vi "Publish.vi"(6 "Publish Time":timestamp, 8 "error in (no error)":errorcluster, 9 "Data to Publish":variant, 10 "Datum Name":string, 11 "Mediator in":refnum<class "Mediator.lvclass">) -> (0 "error out":errorcluster, 3 "Mediator out":refnum<class "Mediator.lvclass">)   [LabVIEW 2015, in "Mediator.lvlib" / "Mediator.lvclass"]
doc: "<License>\nCopyright © 2017 Composed Systems, LLC | All rights reserved\nwww.composed.io\n\nAuthor: Ethan Stern <ethan.stern@composed.io>\n\nThis software is provided \"AS IS\" WITHOUT WARRANTIES, either express or implied, AND IS FOR EDUCATIONAL PURPOSES ONLY.\n</License>"
uses:
  Mediator.lvclass
  Mediator.lvclass/Mediator.ctl
  Topic Messages/Notify Subscribers Msg/Notify Subscribers Msg.lvclass/Notify Subscribers Msg.ctl
  <vilib>/ActorFramework/Message Enqueuer/Message Enqueuer.lvclass/Message Enqueuer.ctl
  <vilib>/ActorFramework/Message Enqueuer/Enqueue.vi
  <vilib>/ActorFramework/Message Priority Queue/Priority Enqueue.vi
  Topic Messages/Notify Subscribers Msg/Notify Subscribers Msg.lvclass
  TopicLookupTable/TopicLookupTable.lvclass
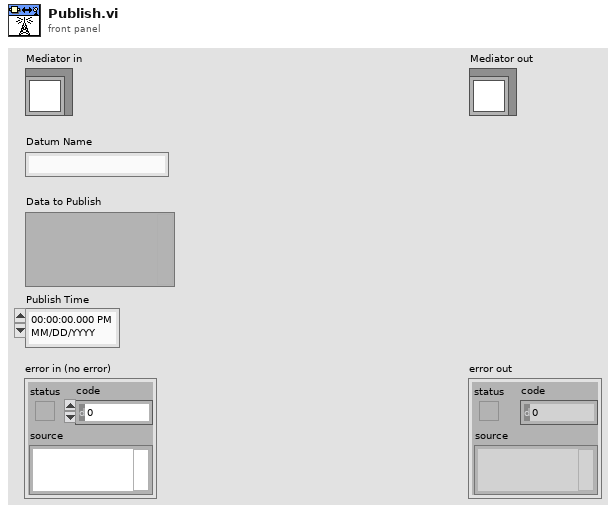
[diagram p1: front panel]
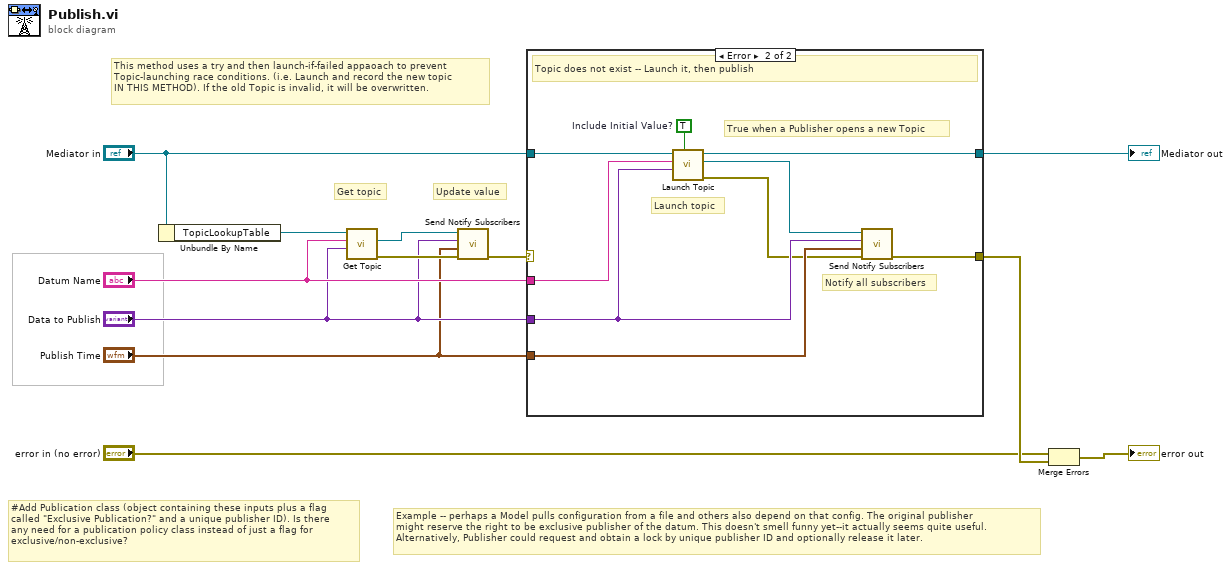
[diagram p0: block diagram]
diagram:
  # "Example -- perhaps a Model pulls configuration from a file and others also depend on that config. The original publisher\nmight reserve the right to be exclusive publisher of the datum. This doesn't smell funny yet--it actually seems quite useful.\nAlternatively, Publisher could request and obtain a lock by unique publisher ID and optionally release it later."
  # "#Add Publication class (object containing these inputs plus a flag \ncalled \"Exclusive Publication?\" and a unique publisher ID). Is there\nany need for a publication policy class instead of just a flag for\nexclusive/non-exclusive?"
  # "This method uses a try and then launch-if-failed appaoach to prevent\nTopic-launching race conditions. (i.e. Launch and record the new topic\nIN THIS METHOD). If the old Topic is invalid, it will be overwritten."
  # "Update value"
  # "Get topic"
  n1 = Unbundle By Name("Mediator in") -> ("TopicLookupTable"=w1:refnum<data-value>)
  n2 = call "Get Topic.vi"("Topic Type"="Data to Publish", "Topic Name"="Datum Name", "TopicLookupTable"=w1) -> ("error out"=w9:errorcluster, "Topic Enqueuer"=w12:refnum<class "Message Enqueuer.lvclass">)  [unwired: 6 in, 1 out]
  n3 = call "Send Notify Subscribers.vi"("error in (no error)"=w9, "Publish Time"="Publish Time", "Topic Data"="Data to Publish", "Message Enqueuer"=w12) -> ("error out"=w11:errorcluster)  [unwired: 6 in, 1 out]
  n4 = case shown="Error" w11 {
    selector: w11 -> [w13 _]
    tunnel: "Mediator in" -> [w14 w23]
    tunnel: [w14 w20] -> w7
    tunnel: "Datum Name" -> [_ w18]
    tunnel: "Data to Publish" -> [_ w17]
    tunnel: [w13 w22] -> w10
    tunnel: "Publish Time" -> [_ w21]
    frame No Error {
      # "Topic exists -- Publish OK"
    }
    frame Error {
      w15 = TRUE  # Include Initial Value?
      # "True when a Publisher opens a new Topic"
      # "Launch topic"
      # "Notify all subscribers"
      # "Topic does not exist -- Launch it, then publish"
      n5 = call "Launch Topic.vi"("Include Initial Value? (F)"=w15, "Type"=w17, "Datum Name"=w18, "Mediator in"=w23) -> ("error out"=w16:errorcluster, "New Topic Enqueuer"=w19:refnum<class "Message Enqueuer.lvclass">, "Mediator out"=w20:refnum<class "Mediator.lvclass">)  [unwired: 5 in]
      n6 = call "Send Notify Subscribers.vi"("error in (no error)"=w16, "Publish Time"=w21, "Topic Data"=w17, "Message Enqueuer"=w19) -> ("error out"=w22:errorcluster)  [unwired: 6 in, 1 out]
    }
  }
  "Mediator out" <- w7
  n7 = Merge Errors("error in (no error)", w10) -> (→"error out":errorcluster)
